vi "Write Configuration Version.vi"(8 "error in (no error)":errorcluster, 10 "Configuration Version":T1, 11 "Configuration Session in":refnum<class "Configuration Session.lvclass">) -> (0 "error out":errorcluster, 3 "Configuration Session out":refnum<class "Configuration Session.lvclass">)   [LabVIEW 2017, in "DSF Core.lvlib" / "Configuration Session.lvclass"]
doc: "Writes a value to a key in a specified section of the configuration data identified by <B>dsf refnum</B>. This VI modifies data in memory. To write data to disk, use the Close Config Data VI. Wire data to the <B>value</B> input to determine the polymorphic instance to use or manually select the instance."
uses:
  Configuration Session.lvclass
  Public/Controls/DSF Version Info.ctl
  Configuration Session.lvclass/Configuration Session.ctl
  DSF Core.lvlib
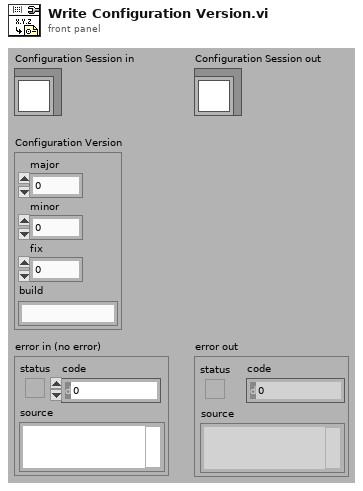
[diagram p1: front panel]
types:
  T1 = typedef "DSF Core.lvlib/DSF Version Info.ctl" = cluster{"major":u32, "minor":u32, "fix":u32, "build":string}
  T2 = typedef "DSF Core.lvlib/Configuration Session.lvclass/DSF Config Data Ref.ctl" = refnum<data-value>
  T3 = typedef "DSF Core.lvlib/Configuration Session.lvclass/DSF Config Data.ctl" = cluster{"dsf configuration":T4, "path":path, "dirty":bool}
  T4 = typedef "DSF Core.lvlib/Configuration Session.lvclass/Internal DSF Configuration.ctl" = cluster{"dsfversion":T1, "version":T1, "plugins":T5[], "groups":T8[], "transfers":T10[], "channels":T12[], "settings":T14[]}
  T5 = typedef "DSF Core.lvlib/Configuration Session.lvclass/Internal DSF Plugin with ID.ctl" = cluster{"id":string, "values":T6}
  T6 = typedef "DSF Core.lvlib/Configuration Session.lvclass/Internal DSF Plugin Info.ctl" = cluster{"type":string, "timing":T7, "group ids":string[], "settings id":string, "thread count":i32}
  T7 = typedef "DSF Core.lvlib/DSF Timing Info.ctl" = cluster{"priority":u64, "decimation":u64, "offset":u64}
  T8 = typedef "DSF Core.lvlib/Configuration Session.lvclass/Internal DSF Group with ID.ctl" = cluster{"id":string, "values":T9}
  T9 = typedef "DSF Core.lvlib/Configuration Session.lvclass/Internal DSF Group Info.ctl" = cluster{"direction":i32, "timing":T7, "transfer ids":string[], "settings id":string}
  T10 = typedef "DSF Core.lvlib/Configuration Session.lvclass/Internal DSF Transfer with ID.ctl" = cluster{"id":string, "values":T11}
  T11 = typedef "DSF Core.lvlib/Configuration Session.lvclass/Internal DSF Transfer Info.ctl" = cluster{"byte order":i32, "channel ids":string[], "settings id":string}
  T12 = typedef "DSF Core.lvlib/Configuration Session.lvclass/Internal DSF Channel with ID.ctl" = cluster{"id":string, "values":T13}
  T13 = typedef "DSF Core.lvlib/Configuration Session.lvclass/Internal DSF Channel Info.ctl" = cluster{"count":u64, "buffer offset":u64, "data type":i32, "settings id":string}
  T14 = typedef "DSF Core.lvlib/Configuration Session.lvclass/Internal DSF Settings with ID.ctl" = cluster{"id":string, "values":T15}
  T15 = typedef "DSF Core.lvlib/Configuration Session.lvclass/Internal DSF Settings Info.ctl" = cluster{"key":string, "value":string}[]
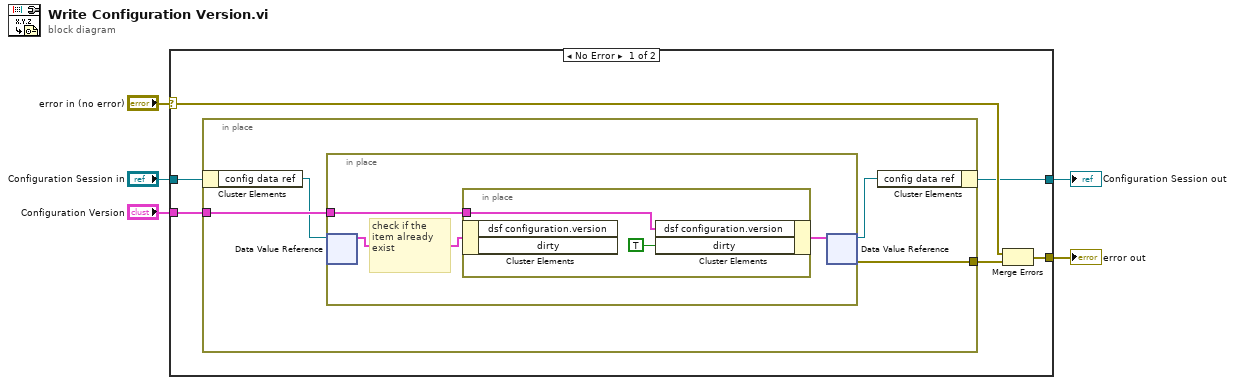
[diagram p0: block diagram]
diagram:
  n1 = case shown="No Error" "error in (no error)" {
    selector: "error in (no error)" -> [w9 w22]
    tunnel: [w8 w22] -> w4
    tunnel: [w6 w21] -> w1
    tunnel: "Configuration Version" -> [w11 _]
    tunnel: "Configuration Session in" -> [w7 w21]
    frame No Error {
      n2 = in-place {
        in-place-border: w11 -> [w15]
        in-place-border: [w14] -> w10
        n3 = in-place-cluster #1(w7) -> ("config data ref"=w13:T2)
        n4 = in-place {
          in-place-border: w15 -> [w18]
          # "check if the item already exist"
          n5 = in-place-dvr #2(w13) -> (w17:T3)  [unwired: 1 out]
          n6 = in-place {
            in-place-border: w18 -> [w19]
            n7 = in-place-cluster #3(w17) -> ()  [unwired: 2 out]
            n8 = in-place-cluster #3("dsf configuration.version"=w19, "dirty"=TRUE) -> (w16:T3)
          }
          n9 = in-place-dvr #2(w16) -> (w12:T2, w14:errorcluster)
        }
        n10 = in-place-cluster #1("config data ref"=w12) -> (w6:refnum<class "Configuration Session.lvclass">)
      }
      n11 = Merge Errors(w9, w10) -> (w8:errorcluster)
    }
    frame Error {
    }
  }
  "error out" <- w4
  "Configuration Session out" <- w1
